vi "Triekselfy Project.vi"() -> ()   [LabVIEW 2021]
panel:
  out "Progress":sgl(slide) scale=0.0..1.0
  out "Name":string
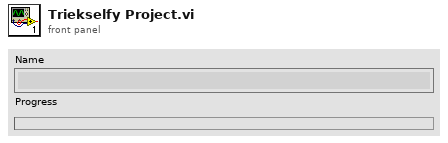
[diagram p1: front panel]
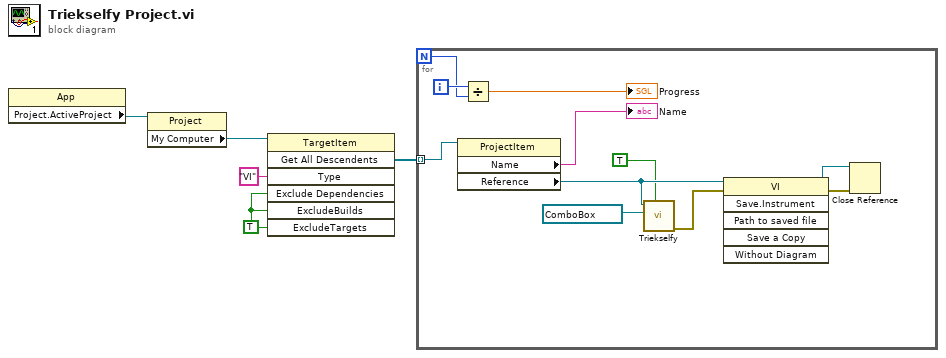
[diagram p0: block diagram]
diagram:
  w2 = TRUE ("ExcludeTargets")
  n1 = property class="App"() -> ("Project.ActiveProject"=w5:refnum<vi>)  [unwired: 2 in, 2 out]
  n2 = property class="Project"(reference=w5) -> ("My Computer"=w4:refnum<vi>)  [unwired: 1 in, 2 out]
  n3 = invoke class="TargetItem" method="Get All Descendents"(reference=w4, "Type"="VI", "Exclude Dependencies"=w2, "ExcludeBuilds"=w2, "ExcludeTargets"=w2) -> ("All Descendents"=w1:refnum<vi>[])  [unwired: 2 in, 6 out]
  n4 = for {
    N -> [w7]
    tunnel: w1 -> [w14] mode=indexing
    i -> [w8]
    n5 = property class="ProjectItem"(reference=w14) -> ("Name"=→"Name":string, "Reference"=w12:refnum<vi>)  [unwired: 1 in, 2 out]
    n6 = Divide(x=w8, y=w7) -> (x/y=→"Progress":dbl)
    n7 = call <resource>:"Triekselfy.vi"("Shift Pressed?"=TRUE, "QD Combo Box Ref"=refnum<vi> refnum, "QD Launch VI Ref"=w12) -> ("error out"=w15:errorcluster)  [unwired: 7 in, 1 out]
    n8 = invoke class="VI" method="Save.Instrument"(reference=w12, error in=w15) -> (reference out=w13:refnum<vi>, error out=w16:errorcluster)  [unwired: 4 in, 4 out]
    n9 = Close Reference(reference=w13, error in (no error)=w16) -> ()  [unwired: 1 out]
  }
